vi "setParameters.vi"(10 "Parameters":T1, 11 "ApplyAberrationByBendingModesCommand in":refnum<class "ApplyAberrationByBendingModesCommand.lvclass">) -> (3 "ApplyAberrationByBendingModesCommand out":refnum<class "ApplyAberrationByBendingModesCommand.lvclass">)   [LabVIEW 2016, in "ApplyAberrationByBendingModesCommand.lvclass"]
uses:
  ApplyAberrationByBendingModesCommand.lvclass
  DataTypes/Topics/CommandApplyAberrationByBendingModes.ctl
  DataTypes/Topics/Parts/CommandId.ctl
  ApplyAberrationByBendingModesCommand.lvclass/ApplyAberrationByBendingModesCommand.ctl
  DataTypes/Topics/M1M3SupportTopics.lvlib
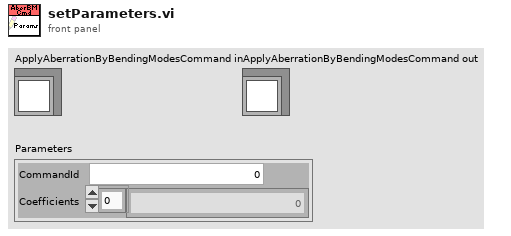
[diagram p1: front panel]
types:
  T1 = typedef "M1M3SupportTopics.lvlib/CommandApplyAberrationByBendingModes.ctl" = cluster{"CommandId":T2, "Coefficients":dbl[]}
  T2 = typedef "M1M3SupportTopics.lvlib/CommandId.ctl" = i32
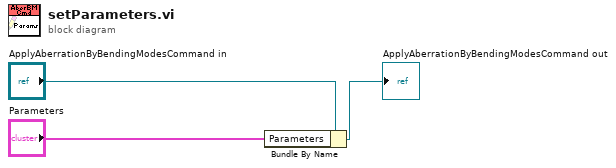
[diagram p0: block diagram]
diagram:
  n1 = Bundle By Name(cluster="ApplyAberrationByBendingModesCommand in", "Parameters"="Parameters") -> (→"ApplyAberrationByBendingModesCommand out":refnum<class "ApplyAberrationByBendingModesCommand.lvclass">)
